vi "TLMB_Get_Single_Fault_Snapshot.vi"(0 "GEA2 Reference In":refnum<k24>, 5 "Standalone?":bool, 7 "Snapshot Selection":T2, 11 "Error In":errorcluster) -> (4 "GEA2 Reference Out":refnum<k24>, 6 "Fault Snapshots":T1, 15 "Error Out":errorcluster)   [LabVIEW 2021, in "TLMB.lvlib"]
uses:
  Projects/TLMB.lvlib
  subVIs/Snap_Selection.ctl
  D:/Common/LabVIEW GEA2 Toolkit/source/GEA3 DLL Source/GeaCommunication.dll
  Common/LabVIEW GEA2 Toolkit/source/GEA3 DLL Source/GeaCommunication.dll
  subVIs/Snap_Input.ctl
  Common/LabVIEW GEA2 Toolkit/GEA3/type defs/Source_Destination.ctl
  Common/LabVIEW GEA2 Toolkit/GEA3/type defs/ERD Read Data In.ctl
  Common/LabVIEW GEA2 Toolkit/GEA3/library/GEA2_Toolkit.lvlib
panel:
  out "ERD Number":string
  out "ERD Data":string
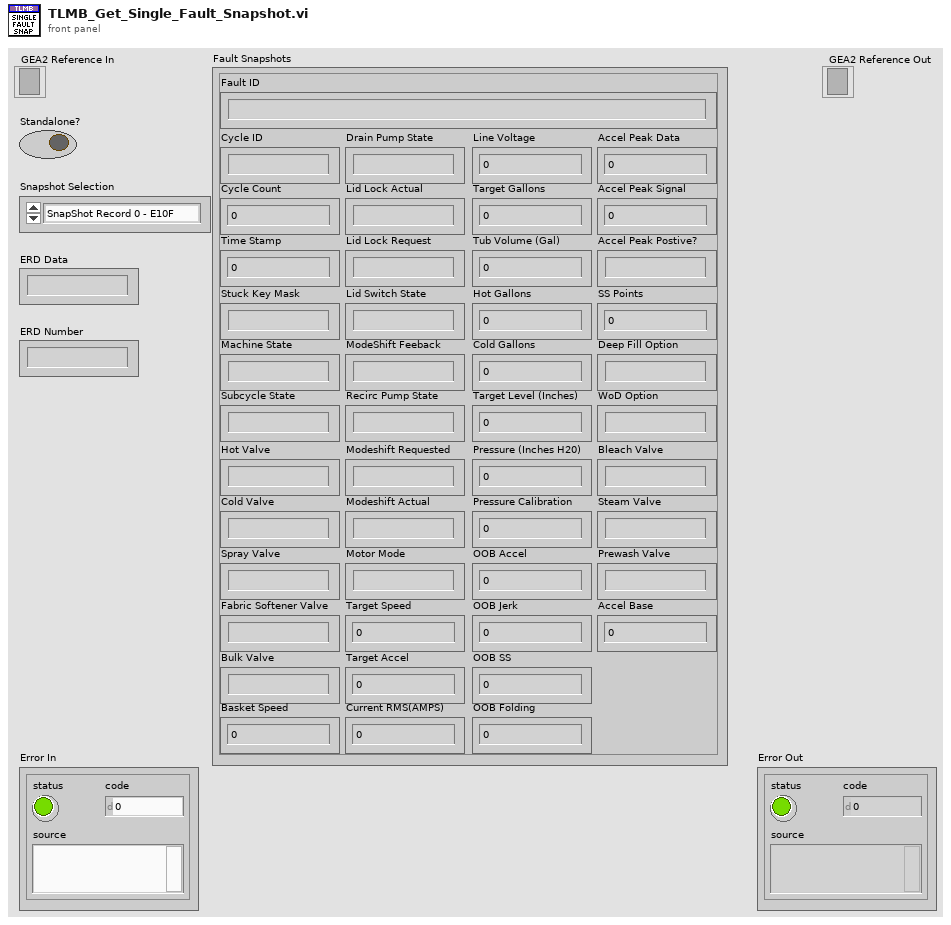
[diagram p1: front panel]
types:
  T1 = typedef "TLMB.lvlib/Snap_Input.ctl" = cluster{"Fault ID":string, "Cycle Count":u32, "Cycle ID":string, "Time Stamp":u32, "Stuck Key Mask":string, "Machine State":string, "Subcycle State":string, "Hot Valve":string, "Cold Valve":string, "Spray Valve":string, "Fabric Softener Valve":string, "Bulk Valve":string, "Drain Pump State":string, "Lid Lock Actual":string, "Lid Lock Request":string, "Lid Switch State":string, "ModeShift Feeback":string, "Recirc Pump State":string, "Modeshift Requested":string, "Modeshift Actual":string, "Motor Mode":string, "Target Speed":u16, "Target Accel":u16, "Current RMS(AMPS)":dbl, "Line Voltage":dbl, "Target Gallons":dbl, "Tub Volume (Gal)":dbl, "Hot Gallons":dbl, "Cold Gallons":dbl, "Target Level (Inches)":dbl, "Pressure (Inches H20) ":dbl, "Pressure Calibration":dbl, "OOB Accel":i32, "OOB Jerk":i32, "OOB SS":i32, "OOB Folding":i32, "Accel Peak Data":i16, "Accel Peak Signal":u8, "Accel Peak Postive?":string, "SS Points":u8, "Deep Fill Option":string, "WoD Option":string, "Basket Speed":u16, "Bleach Valve":string, "Steam Valve":string, "Prewash Valve":string, "Accel Base":i16}
  T2 = typedef "TLMB.lvlib/Snap_Selection.ctl" = enum16{"SnapShot Record 0 - E10F", "Snapshot Record 1 - E110", "Snapshot Record 2 - E111", "Snapshot Record 3 - E112", "Snapshot Record 4 - E113", "Snapshot Record 5 - E114", "Snapshot Record 6 - E115", "Snapshot Record 7 - E116", "Snapshot Record 8 - E117", "Snapshot Record 9 - E118"}
  T3 = typedef "Source_Destination.ctl" = cluster{"Source":u8, "Destination":u8}
  T4 = typedef "ERD Read Data In.ctl" = cluster{"ERD Number":u16, "Data Type":enum16{"string", "boolean", "uint8_t", "uint16_t", "uint32_t", "uint64_t", "int8_t", "int16_t", "int32_t", "int64_t"}}
  T5 = typedef "ERD Read Data Out.ctl" = cluster{"ERD Number":u16, "Data":string}
  T6 = cluster{"ERD Data Out[0]":T5, "ERD Data Out[1]":T5, "ERD Data Out[2]":T5, "ERD Data Out[3]":T5, "ERD Data Out[4]":T5, "ERD Data Out[5]":T5, "ERD Data Out[6]":T5, "ERD Data Out[7]":T5, "ERD Data Out[8]":T5}
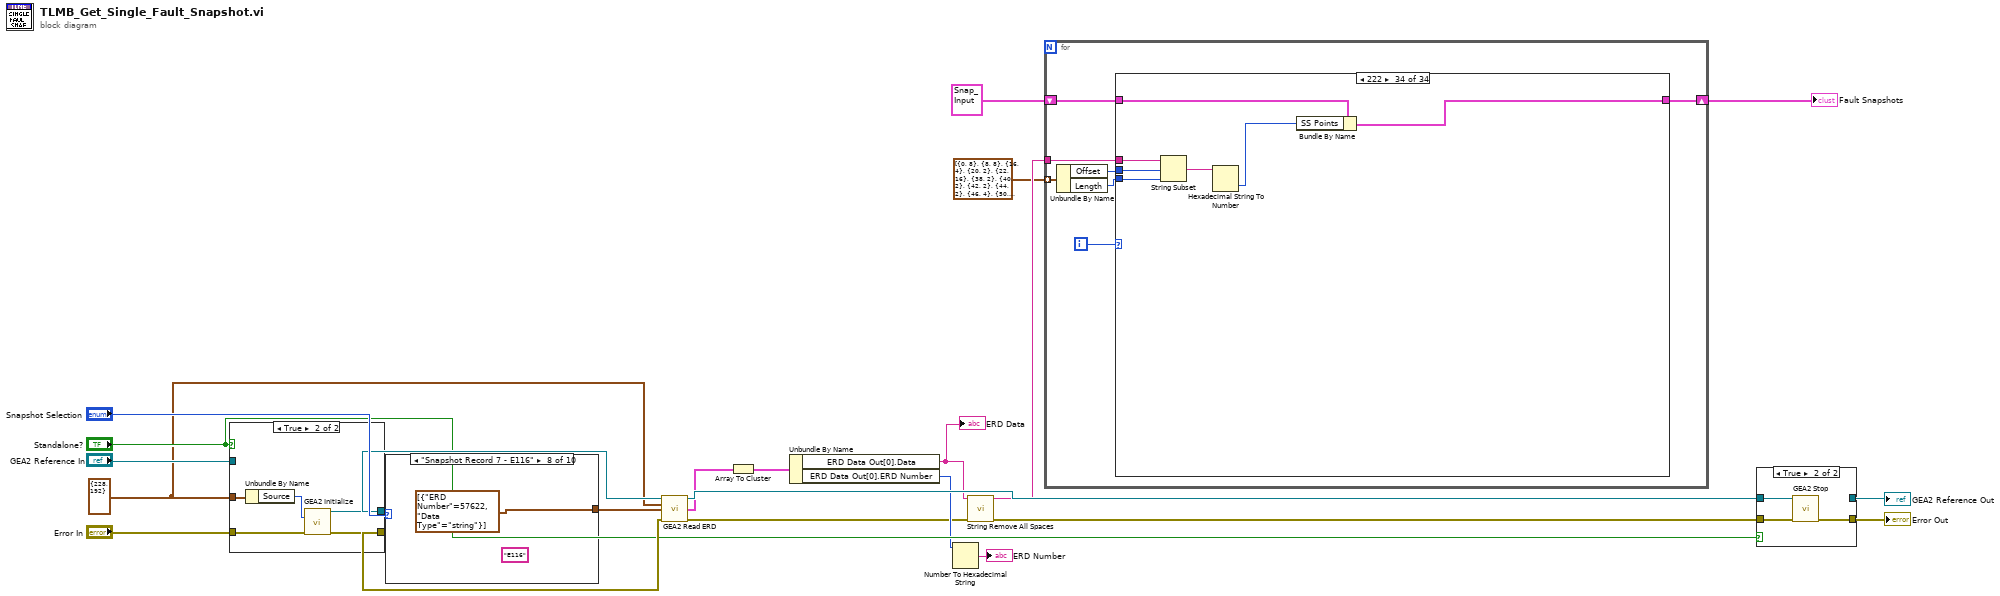
[diagram p0: block diagram]
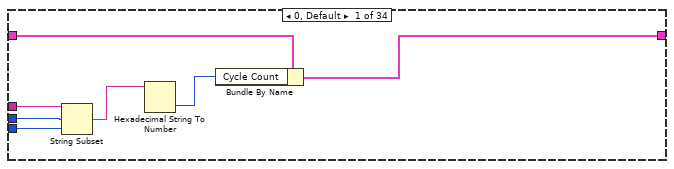
[diagram p2: hidden frame]
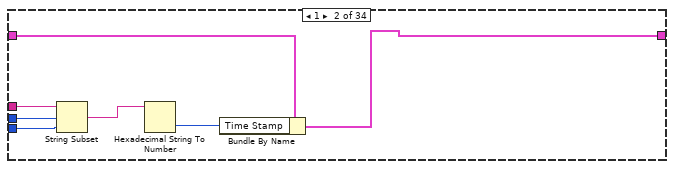
[diagram p3: hidden frame]
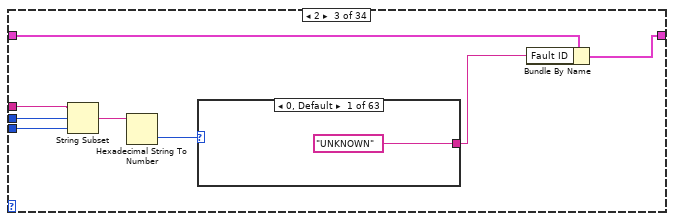
[diagram p4: hidden frame]
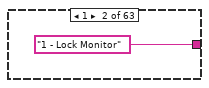
[diagram p5: hidden frame]
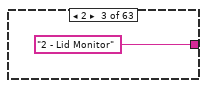
[diagram p6: hidden frame]
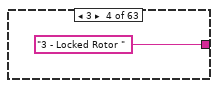
[diagram p7: hidden frame]
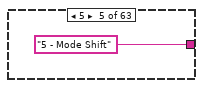
[diagram p8: hidden frame]
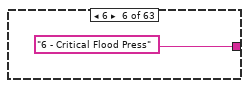
[diagram p9: hidden frame]
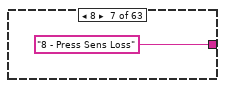
[diagram p10: hidden frame]
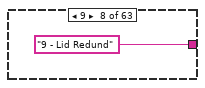
[diagram p11: hidden frame]
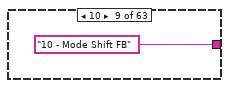
[diagram p12: hidden frame]
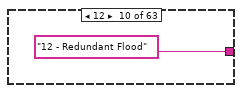
[diagram p13: hidden frame]
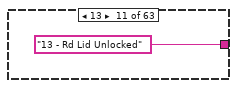
[diagram p14: hidden frame]
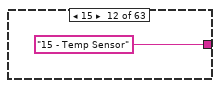
[diagram p15: hidden frame]
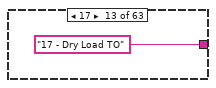
[diagram p16: hidden frame]
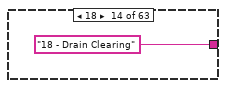
[diagram p17: hidden frame]
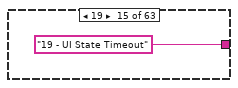
[diagram p18: hidden frame]
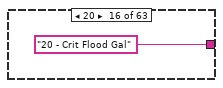
[diagram p19: hidden frame]
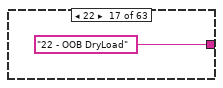
[diagram p20: hidden frame]
diagram:
  w13 = T3 {"Source"=228, "Destination"=192} ("GEA Inputs")
  n1 = case shown="True" "Standalone?" {
    tunnel: "Error In" -> [w23 w29]
    tunnel: [w23 w28] -> w17
    tunnel: "GEA2 Reference In" -> [w24 _]
    tunnel: [w24 w27] -> w18
    tunnel: w13 -> [_ w25]
    frame False {
    }
    frame True {
      n2 = Unbundle By Name(w25) -> ("Source"=w26:u8)
      n3 = call "GEA2 Initialize.vi"("Source Address"=w26, "error in"=w29) -> ("GEA2 Reference Out"=w27:refnum<k24>, "error out"=w28:errorcluster)  [unwired: 11 in, 1 out]
    }
  }
  n4 = case shown="\"Snapshot Record 7 - E116\"" "Snapshot Selection" {
    tunnel: [T4[] [{"ERD Number"=57615, "Data Type"=enum."string"}] ("Read ERD List") T4[] [{"ERD Number"=57616, "Data Type"=enum."string"}] ("Read ERD List") T4[] [{"ERD Number"=57617, "Data Type"=enum."string"}] ("Read ERD List") T4[] [{"ERD Number"=57618, "Data Type"=enum."string"}] ("Read ERD List") T4[] [{"ERD Number"=57619, "Data Type"=enum."string"}] ("Read ERD List") T4[] [{"ERD Number"=57620, "Data Type"=enum."string"}] ("Read ERD List") T4[] [{"ERD Number"=57621, "Data Type"=enum."string"}] ("Read ERD List") T4[] [{"ERD Number"=57622, "Data Type"=enum."string"}] ("Read ERD List") T4[] [{"ERD Number"=57623, "Data Type"=enum."string"}] ("Read ERD List") T4[] [{"ERD Number"=57624, "Data Type"=enum."string"}] ("Read ERD List")] -> w21
    frame "SnapShot Record 0 - E10F", Default {
      (unwired) "E10F"
    }
    frame "Snapshot Record 1 - E110" {
      (unwired) "E110"
    }
    frame "Snapshot Record 2 - E111" {
      (unwired) "E111"
    }
    frame "Snapshot Record 3 - E112" {
      (unwired) "E112"
    }
    frame "Snapshot Record 4 - E113" {
      (unwired) "E113"
    }
    frame "Snapshot Record 5 - E114" {
      (unwired) "E114"
    }
    frame "Snapshot Record 6 - E115" {
      (unwired) "E115"
    }
    frame "Snapshot Record 7 - E116" {
      (unwired) "E116"
    }
    frame "Snapshot Record 8 - E117" {
      (unwired) "E117"
    }
    frame "Snapshot Record 9 - E118" {
      (unwired) "E118"
    }
  }
  n5 = call "GEA2 Read ERD.vi"("GEA2 Reference In"=w18, "GEA Inputs"=w13, "Read ERD List"=w21, "Error In"=w17) -> ("GEA2 Reference Out"=w16:refnum<k24>, "ERD Data Out"=w12:T5[], "Error Out"=w7:errorcluster)  [unwired: 8 in, 1 out]
  n6 = Array To Cluster(array=w12) -> (cluster=w11:T6)
  n7 = Unbundle By Name(w11) -> ("ERD Data Out[0].Data"=w8:string, "ERD Data Out[0].ERD Number"=w10:u16)
  "ERD Data" <- w8
  n8 = Number To Hexadecimal String(2:w10) -> (0:→"ERD Number":string)  [unwired: 1 in]
  n9 = call "String Remove All Spaces.vi"("Input String"=w8, "error in (no error)"=w7) -> ("Spaces Removed"=w4:string, "error out"=w6:errorcluster)  [unwired: 12 in]
  n10 = for {
    tunnel: w4 -> [w46]
    shift-right: [w44] -> w1
    shift-left: T1 {"Fault ID"="", "Cycle Count"=0, "Cycle ID"="", "Time Stamp"=0, "Stuck Key Mask"="", "Machine State"="", "Subcycle State"="", "Hot Valve"="", "Cold Valve"="", "Spray Valve"="", "Fabric Softener Valve"="", "Bulk Valve"="", "Drain Pump State"="", "Lid Lock Actual"="", "Lid Lock Request"="", "Lid Switch State"="", "ModeShift Feeback"="", "Recirc Pump State"="", "Modeshift Requested"="", "Modeshift Actual"="", "Motor Mode"="", "Target Speed"=0, "Target Accel"=0, "Current RMS(AMPS)"=0.0, "Line Voltage"=0.0, "Target Gallons"=0.0, "Tub Volume (Gal)"=0.0, "Hot Gallons"=0.0, "Cold Gallons"=0.0, "Target Level (Inches)"=0.0, "Pressure (Inches H20) "=0.0, "Pressure Calibration"=0.0, "OOB Accel"=0, "OOB Jerk"=0, "OOB SS"=0, "OOB Folding"=0, "Accel Peak Data"=0, "Accel Peak Signal"=0, "Accel Peak Postive?"="", "SS Points"=0, "Deep Fill Option"="", "WoD Option"="", "Basket Speed"=0, "Bleach Valve"="", "Steam Valve"="", "Prewash Valve"="", "Accel Base"=0} ("input cluster") -> [w45]
    tunnel: cluster{"Offset":i32, "Length":i32}[] [{"Offset"=0, "Length"=8}, {"Offset"=8, "Length"=8}, {"Offset"=16, "Length"=4}, {"Offset"=20, "Length"=2}, {"Offset"=22, "Length"=16}, {"Offset"=38, "Length"=2}, {"Offset"=40, "Length"=2}, {"Offset"=42, "Length"=2}, {"Offset"=44, "Length"=2}, {"Offset"=46, "Length"=4}, {"Offset"=50, "Length"=4}, {"Offset"=54, "Length"=4}, {"Offset"=58, "Length"=4}, {"Offset"=62, "Length"=8}, {"Offset"=70, "Length"=8}, {"Offset"=78, "Length"=8}, {"Offset"=86, "Length"=8}, {"Offset"=94, "Length"=8}, {"Offset"=102, "Length"=8}, {"Offset"=110, "Length"=4}, {"Offset"=114, "Length"=2}, {"Offset"=116, "Length"=2}, {"Offset"=118, "Length"=4}, {"Offset"=104, "Length"=8}, {"Offset"=112, "Length"=8}, {"Offset"=120, "Length"=8}, {"Offset"=128, "Length"=8}, {"Offset"=136, "Length"=8}, {"Offset"=144, "Length"=4}, {"Offset"=148, "Length"=4}, {"Offset"=152, "Length"=2}, {"Offset"=154, "Length"=2}, {"Offset"=156, "Length"=2}, {"Offset"=158, "Length"=2}] -> [w41] mode=indexing
    i -> [w43]
    n11 = Unbundle By Name(w41) -> ("Offset"=w42:i32, "Length"=w40:i32)
    n12 = case shown="222" w43 {
      tunnel: w46 -> [w51 w60 w67 w139 w188 w211 w231 w264 w288 w301 w311 w321 w331 w341 w351 w358 w365 w372 w379 w386 w393 w401 w409 w420 w429 w448 w456 w464 w474 w484 w494 w520 w543 w557]
      tunnel: w42 -> [w50 w59 w66 w138 w187 w210 w230 w263 w287 w300 w310 w320 w330 w340 w350 w357 w364 w371 w378 w385 w392 w400 w408 w419 w428 w447 w455 w463 w473 w483 w493 w519 w542 w556]
      tunnel: w40 -> [w49 w58 w65 w137 w186 w209 w229 w262 w286 w299 w309 w319 w329 w339 w349 w356 w363 w370 w377 w384 w391 w399 w407 w418 w427 w446 w454 w462 w472 w482 w492 w518 w541 w555]
      tunnel: w45 -> [w53 w57 w68 w136 w190 w213 w228 w266 w290 w303 w313 w323 w333 w343 w353 w360 w367 w374 w381 w388 w395 w403 w412 w417 w431 w450 w458 w466 w476 w486 w496 w522 w545 w559]
      tunnel: [w52 w56 w64 w135 w189 w212 w227 w265 w289 w302 w312 w322 w332 w342 w352 w359 w366 w373 w380 w387 w394 w402 w411 w416 w430 w449 w457 w465 w475 w485 w495 w521 w544 w558] -> w44
      frame 0, Default {
        n13 = String Subset(string=w51, offset (0)=w50, length (rest)=w49) -> (substring=w48:string)
        n14 = Hexadecimal String To Number(string=w48) -> (number=w47:u32)  [unwired: 2 in, 1 out]
        n15 = Bundle By Name(cluster=w53, "Cycle Count"=w47) -> (w52:T1)
      }
      frame 1 {
        n16 = String Subset(string=w60, offset (0)=w59, length (rest)=w58) -> (substring=w55:string)
        n17 = Hexadecimal String To Number(string=w55) -> (number=w54:u32)  [unwired: 2 in, 1 out]
        n18 = Bundle By Name(cluster=w57, "Time Stamp"=w54) -> (w56:T1)
      }
      frame 2 {
        n19 = String Subset(string=w67, offset (0)=w66, length (rest)=w65) -> (substring=w63:string)
        n20 = Hexadecimal String To Number(string=w63) -> (number=w62:u32)  [unwired: 2 in, 1 out]
        n21 = case shown="0, Default" w62 {
          tunnel: ["UNKNOWN" "1 - Lock Monitor" "2 - Lid Monitor" "3 - Locked Rotor " "5 - Mode Shift" "6 - Critical Flood Press" "8 - Press Sens Loss" "9 - Lid Redund" "10 - Mode Shift FB" "12 - Redundant Flood" "13 - Rd Lid Unlocked" "15 - Temp Sensor" "17 - Dry Load TO" "18 - Drain Clearing" "19 - UI State Timeout" "20 - Crit Flood Gal" "22 - OOB DryLoad" "23 - Crit LidLock: Can't Lock" "24 - Lid Logic" "25 - Press Sens Dropout" "26 - OOB Redist" "27 - Water Access" "28 - ADC Knob" "29 - Suds Lock" "30 - Stuck Button" "31 - OOB Fallback" "32 - Crit LidLock: Can't Unlock" "33 - Crit Inv Reset in Run" "34 - Inv Boot Failure" "35 - Accel Chip Comm Failure" "41 - Inv LGBT Temp Sensor" "42 - Inv LGBT Temp Overheat" "43 - Inv Gate Driver" "44 - Inv Gate Crit Over Current" "45 - Inv DC Bus Voltage Crit" "46 - Inv MC API Ver" "47 - Inv MC Command Crit" "48 - Inv Heatsink Temp" "49 - Inv Motor Over Temp" "50 - Inv Crit Low Voltage" "51 - Inv Crit Locked Rotor" "52 - Inv Motor Over Temp" "100 - Accelrmtr Comm" "101 - Max Fill Pressure" "102 - Clock Mon" "103 - LidLock Failure" "104 - Adaptive Drain" "105 - Max Fill Volume" "106 - Target Spin Speed Timeout" "107 - Target Spin Speed Dropout" "108 - UI-MC Heatbeat Timeout" "109 - Event Seq Overflow" "111 - Inv Reset in Cycle Run" "114 - Utility Micro Comm" "115 - Accel Heartbeat" "119 - Inv LGBT Temp Overheat" "120 - Inv Gate Over Current" "121 - Inv DC Bus Voltage" "122 - Inv MC Command" "123 - Inv Heatsink Overheat" "124 - Inv Low Voltage" "125 - Inv Locked Rotor" "126 - Phase Fault"] -> w61
          frame 0, Default {
          }
          frame 1 {
          }
          frame 2 {
          }
          frame 3 {
          }
          frame 5 {
          }
          frame 6 {
          }
          frame 8 {
          }
          frame 9 {
          }
          frame 10 {
          }
          frame 12 {
          }
          frame 13 {
          }
          frame 15 {
          }
          frame 17 {
          }
          frame 18 {
          }
          frame 19 {
          }
          frame 20 {
          }
          frame 22 {
          }
          frame 23 {
          }
          frame 24 {
          }
          frame 25 {
          }
          frame 26 {
          }
          frame 27 {
          }
          frame 28 {
          }
          frame 29 {
          }
          frame 30 {
          }
          frame 31 {
          }
          frame 32 {
          }
          frame 33 {
          }
          frame 34 {
          }
          frame 35 {
          }
          frame 41 {
          }
          frame 42 {
          }
          frame 43 {
          }
          frame 44 {
          }
          frame 45 {
          }
          frame 46 {
          }
          frame 47 {
          }
          frame 48 {
          }
          frame 49 {
          }
          frame 50 {
          }
          frame 51 {
          }
          frame 52 {
          }
          frame 100 {
          }
          frame 101 {
          }
          frame 102 {
          }
          frame 103 {
          }
          frame 104 {
          }
          frame 105 {
          }
          frame 106 {
          }
          frame 107 {
          }
          frame 108 {
          }
          frame 109 {
          }
          frame 111 {
          }
          frame 114 {
          }
          frame 115 {
          }
          frame 119 {
          }
          frame 120 {
          }
          frame 121 {
          }
          frame 122 {
          }
          frame 123 {
          }
          frame 124 {
          }
          frame 125 {
          }
          frame 126 {
          }
        }
        n22 = Bundle By Name(cluster=w68, "Fault ID"=w61) -> (w64:T1)
      }
      frame 3 {
        n23 = String Subset(string=w139, offset (0)=w138, length (rest)=w137) -> (substring=w134:string)
        n24 = Hexadecimal String To Number(string=w134) -> (number=w133:u32)  [unwired: 2 in, 1 out]
        n25 = case shown="0, Default" w133 {
          tunnel: ["0 - NotDefined" "1 - BasketClean" "2 - DrainAndSpin" "3 - QuickRinse" "4 - BulkyItems" "5 - Sanitize" "6 - TowelsSheets" "8 - Normal_Mixedload" "9 - Whites" "10 - DarkColors" "11 - Jeans" "12 - HandWash" "13 - Delicates" "14 - SpeedWash" "15 - HeavyDuty" "16 - Allergen" "17 - PowerClean" "18 - RinseSpin" "19 - SingleItemWash" "20 - Colors" "21 - ColdWash" "22 - WaterOnDemand" "23 - TubClean" "24 - CasualsWithSteam" "25 - StainWashWithSteam" "26 - DeepClean" "27 - NotUsed_Start" "127 - NotUsed_End" "128 - Cottons" "129 - EasyCare" "130 - ActiveWear" "131 - TimedDry" "132 - DeWrinkle" "133 - QuickAirFluff" "134 - SteamRefresh" "135 - SteamDewrinkle" "136 - SpeedDry" "137 - Mixed" "138 - Quickdry" "139 - Casuals" "140 - Warmup" "141 - EnergySaver" "142 - Antibacterial"] -> w132
          frame 0, Default {
          }
          frame 1 {
          }
          frame 2 {
          }
          frame 3 {
          }
          frame 4 {
          }
          frame 5 {
          }
          frame 6 {
          }
          frame 8 {
          }
          frame 9 {
          }
          frame 10 {
          }
          frame 11 {
          }
          frame 12 {
          }
          frame 13 {
          }
          frame 14 {
          }
          frame 15 {
          }
          frame 16 {
          }
          frame 17 {
          }
          frame 18 {
          }
          frame 19 {
          }
          frame 20 {
          }
          frame 21 {
          }
          frame 22 {
          }
          frame 23 {
          }
          frame 24 {
          }
          frame 25 {
          }
          frame 26 {
          }
          frame 27 {
          }
          frame 127 {
          }
          frame 128 {
          }
          frame 129 {
          }
          frame 130 {
          }
          frame 131 {
          }
          frame 132 {
          }
          frame 133 {
          }
          frame 134 {
          }
          frame 135 {
          }
          frame 136 {
          }
          frame 137 {
          }
          frame 138 {
          }
          frame 139 {
          }
          frame 140 {
          }
          frame 141 {
          }
          frame 142 {
          }
        }
        n26 = Bundle By Name(cluster=w136, "Cycle ID"=w132) -> (w135:T1)
      }
      frame 4 {
        (unwired) ""
        n27 = String Subset(string=w188, offset (0)=w187, length (rest)=w186) -> (substring=w185:string)
        n28 = Hexadecimal String To Number(string=w185) -> (number=w184:u32)  [unwired: 2 in, 1 out]
        n29 = case shown="0, Default" w184 {
          tunnel: ["No Stuck Key" "Smart Dispense" "Delay Wash" "Extra Rinse" "Mycycle" "Spin Button" "Deep Rinse" "Soil Button" "Auto Soak" "Temp Button" "Warm Rinse" "Deep Fill" "Water on Demand" "Power Button" "Start Button"] -> w183
          frame 0, Default {
          }
          frame 1 {
          }
          frame 2 {
          }
          frame 4 {
          }
          frame 8 {
          }
          frame 16 {
          }
          frame 32 {
          }
          frame 64 {
          }
          frame 128 {
          }
          frame 256 {
          }
          frame 512 {
          }
          frame 1024 {
          }
          frame 2048 {
          }
          frame 4096 {
          }
          frame 8192 {
          }
        }
        n30 = Bundle By Name(cluster=w190, "Stuck Key Mask"=w183) -> (w189:T1)
      }
      frame 5 {
        n31 = String Subset(string=w211, offset (0)=w210, length (rest)=w209) -> (substring=w208:string)
        n32 = Hexadecimal String To Number(string=w208) -> (number=w207:u32)  [unwired: 2 in, 1 out]
        n33 = case shown="0, Default" w207 {
          tunnel: ["IDLE" "STANDBY" "RUN" "PAUSE" "EOC" "DSM DELAY RUN" "DELAY RUN" "DELAY PAUSE" "DRAIN TIMEOUT" "CLEAN SPEAK"] -> w206
          frame 0, Default {
          }
          frame 1 {
          }
          frame 2 {
          }
          frame 3 {
          }
          frame 4 {
          }
          frame 5 {
          }
          frame 6 {
          }
          frame 7 {
          }
          frame 8 {
          }
          frame 128 {
          }
        }
        n34 = Bundle By Name(cluster=w213, "Machine State"=w206) -> (w212:T1)
      }
      frame 6 {
        n35 = String Subset(string=w231, offset (0)=w230, length (rest)=w229) -> (substring=w226:string)
        n36 = Hexadecimal String To Number(string=w226) -> (number=w225:u32)  [unwired: 2 in, 1 out]
        n37 = case shown="0, Default" w225 {
          tunnel: ["NONE" "FILL" "SOAK" "WASH" "RINSE" "SPIN" "DRAIN" "EXTRA SPIN" "EXTRA RINSE" "TUMBLE" "LOAD SIZE"] -> w224
          frame 0, Default {
          }
          frame 1 {
          }
          frame 2 {
          }
          frame 3 {
          }
          frame 4 {
          }
          frame 5 {
          }
          frame 6 {
          }
          frame 7 {
          }
          frame 8 {
          }
          frame 9 {
          }
          frame 10 {
          }
        }
        n38 = Bundle By Name(cluster=w228, "Subcycle State"=w224) -> (w227:T1)
      }
      frame 7 {
        n39 = String Subset(string=w264, offset (0)=w263, length (rest)=w262) -> (substring=w260:string)
        n40 = Hexadecimal String To Number(string=w260) -> (number=w261:u32)  [unwired: 2 in, 1 out]
        n41 = Number To Boolean Array(number=w261) -> (Boolean array=w259:bool[])
        n42 = Index Array(array=w259) -> (element #1=w258:bool, element #2=w256:bool, element #3=w255:bool, element #4=w254:bool, element #5=w253:bool, element #6=w245:bool, element #7=w244:bool, element #8=w243:bool)  [unwired: 8 in]
        n43 = case shown="False" w258 {
          tunnel: ["OFF" "ON"] -> w257
          frame False {
          }
          frame True {
          }
        }
        n44 = case shown="False" w256 {
          tunnel: ["OFF" "ON"] -> w252
          frame False {
          }
          frame True {
          }
        }
        n45 = case shown="False" w255 {
          tunnel: ["OFF" "ON"] -> w251
          frame False {
          }
          frame True {
          }
        }
        n46 = case shown="False" w254 {
          tunnel: ["OFF" "ON"] -> w250
          frame False {
          }
          frame True {
          }
        }
        n47 = case shown="False" w253 {
          tunnel: ["OFF" "ON"] -> w249
          frame False {
          }
          frame True {
          }
        }
        n48 = case shown="False" w245 {
          tunnel: ["OFF" "ON"] -> w248
          frame False {
          }
          frame True {
          }
        }
        n49 = case shown="False" w244 {
          tunnel: ["OFF" "ON"] -> w247
          frame False {
          }
          frame True {
          }
        }
        n50 = case shown="False" w243 {
          tunnel: ["OFF" "ON"] -> w246
          frame False {
          }
          frame True {
          }
        }
        n51 = Bundle By Name(cluster=w266, "Hot Valve"=w257, "Cold Valve"=w252, "Spray Valve"=w251, "Fabric Softener Valve"=w250, "Bulk Valve"=w249, "Bleach Valve"=w248, "Steam Valve"=w247, "Prewash Valve"=w246) -> (w265:T1)
      }
      frame 8 {
        n52 = String Subset(string=w288, offset (0)=w287, length (rest)=w286) -> (substring=w285:string)
        n53 = Hexadecimal String To Number(string=w285) -> (number=w284:u32)  [unwired: 2 in, 1 out]
        n54 = case shown="4" w284 {
          tunnel: ["UNKNOWN" "AGITATE" "SPIN" "TRANS TO SPIN" "TRANS TO AGITATE"] -> w283
          frame 0, Default {
          }
          frame 1 {
          }
          frame 2 {
          }
          frame 3 {
          }
          frame 4 {
          }
        }
        n55 = Bundle By Name(cluster=w290, "Modeshift Actual"=w283) -> (w289:T1)
      }
      frame 9 {
        n56 = String Subset(string=w301, offset (0)=w300, length (rest)=w299) -> (substring=w298:string)
        n57 = Hexadecimal String To Number(string=w298) -> (number=w297:u32)  [unwired: 2 in, 1 out]
        n58 = To Unsigned Word Integer(number=w297) -> (unsigned 16bit integer=w296:u16)
        n59 = Bundle By Name(cluster=w303, "Basket Speed"=w296) -> (w302:T1)
      }
      frame 10 {
        n60 = String Subset(string=w311, offset (0)=w310, length (rest)=w309) -> (substring=w308:string)
        n61 = Hexadecimal String To Number(string=w308) -> (number=w305:u32)  [unwired: 2 in, 1 out]
        n62 = To Double Precision Float(number=w305) -> (double precision float=w307:dbl)
        n63 = Divide(x=w307, y=100.0) -> (x/y=w304:dbl)
        n64 = Bundle By Name(cluster=w313, "Tub Volume (Gal)"=w304) -> (w312:T1)
      }
      frame 11 {
        n65 = String Subset(string=w321, offset (0)=w320, length (rest)=w319) -> (substring=w318:string)
        n66 = Hexadecimal String To Number(string=w318) -> (number=w315:u32)  [unwired: 2 in, 1 out]
        n67 = To Double Precision Float(number=w315) -> (double precision float=w317:dbl)
        n68 = Divide(x=w317, y=100.0) -> (x/y=w314:dbl)
        n69 = Bundle By Name(cluster=w323, "Hot Gallons"=w314) -> (w322:T1)
      }
      frame 12 {
        n70 = String Subset(string=w331, offset (0)=w330, length (rest)=w329) -> (substring=w328:string)
        n71 = Hexadecimal String To Number(string=w328) -> (number=w325:u32)  [unwired: 2 in, 1 out]
        n72 = To Double Precision Float(number=w325) -> (double precision float=w327:dbl)
        n73 = Divide(x=w327, y=100.0) -> (x/y=w324:dbl)
        n74 = Bundle By Name(cluster=w333, "Cold Gallons"=w324) -> (w332:T1)
      }
      frame 13 {
        n75 = String Subset(string=w341, offset (0)=w340, length (rest)=w339) -> (substring=w338:string)
        n76 = Hexadecimal String To Number(string=w338) -> (number=w335:u32)  [unwired: 2 in, 1 out]
        n77 = To Double Precision Float(number=w335) -> (double precision float=w337:dbl)
        n78 = Divide(x=w337, y=1000.0) -> (x/y=w334:dbl)
        n79 = Bundle By Name(cluster=w343, "Pressure (Inches H20)"=w334) -> (w342:T1)
      }
      frame 14 {
        n80 = String Subset(string=w351, offset (0)=w350, length (rest)=w349) -> (substring=w348:string)
        n81 = Hexadecimal String To Number(string=w348) -> (number=w345:u32)  [unwired: 2 in, 1 out]
        n82 = To Double Precision Float(number=w345) -> (double precision float=w347:dbl)
        n83 = Divide(x=w347, y=1000.0) -> (x/y=w344:dbl)
        n84 = Bundle By Name(cluster=w353, "Pressure Calibration"=w344) -> (w352:T1)
      }
      frame 15 {
        n85 = String Subset(string=w358, offset (0)=w357, length (rest)=w356) -> (substring=w355:string)
        n86 = Hexadecimal String To Number(string=w355) -> (number=w354:u32)  [unwired: 2 in, 1 out]
        n87 = Bundle By Name(cluster=w360, "OOB Accel"=w354) -> (w359:T1)
      }
      frame 16 {
        n88 = String Subset(string=w365, offset (0)=w364, length (rest)=w363) -> (substring=w362:string)
        n89 = Hexadecimal String To Number(string=w362) -> (number=w361:u32)  [unwired: 2 in, 1 out]
        n90 = Bundle By Name(cluster=w367, "OOB Jerk"=w361) -> (w366:T1)
      }
      frame 17 {
        n91 = String Subset(string=w372, offset (0)=w371, length (rest)=w370) -> (substring=w369:string)
        n92 = Hexadecimal String To Number(string=w369) -> (number=w368:u32)  [unwired: 2 in, 1 out]
        n93 = Bundle By Name(cluster=w374, "OOB SS"=w368) -> (w373:T1)
      }
      frame 18 {
        n94 = String Subset(string=w379, offset (0)=w378, length (rest)=w377) -> (substring=w376:string)
        n95 = Hexadecimal String To Number(string=w376) -> (number=w375:u32)  [unwired: 2 in, 1 out]
        n96 = Bundle By Name(cluster=w381, "OOB Folding"=w375) -> (w380:T1)
      }
      frame 19 {
        n97 = String Subset(string=w386, offset (0)=w385, length (rest)=w384) -> (substring=w383:string)
        n98 = Hexadecimal String To Number(string=w383) -> (number=w382:u32)  [unwired: 2 in, 1 out]
        n99 = Bundle By Name(cluster=w388, "Accel Peak Data"=w382) -> (w387:T1)
      }
      frame 20 {
        n100 = String Subset(string=w393, offset (0)=w392, length (rest)=w391) -> (substring=w390:string)
        n101 = Hexadecimal String To Number(string=w390) -> (number=w389:u32)  [unwired: 2 in, 1 out]
        n102 = Bundle By Name(cluster=w395, "Accel Peak Signal"=w389) -> (w394:T1)
      }
      frame 21 {
        n103 = String Subset(string=w401, offset (0)=w400, length (rest)=w399) -> (substring=w398:string)
        n104 = Hexadecimal String To Number(string=w398) -> (number=w397:u32)  [unwired: 2 in, 1 out]
        n105 = case shown="1" w397 {
          tunnel: ["FALSE" "TRUE"] -> w396
          frame 0, Default {
          }
          frame 1 {
          }
        }
        n106 = Bundle By Name(cluster=w403, "Accel Peak Postive?"=w396) -> (w402:T1)
      }
      frame 22 {
        n107 = String Subset(string=w409, offset (0)=w408, length (rest)=w407) -> (substring=w410:string)
        n108 = Hexadecimal String To Number(string=w410) -> (number=w406:u32)  [unwired: 2 in, 1 out]
        n109 = Bundle By Name(cluster=w412, "Accel Base"=w406) -> (w411:T1)
      }
      frame 23 {
        n110 = String Subset(string=w420, offset (0)=w419, length (rest)=w418) -> (substring=w415:string)
        n111 = Hexadecimal String To Number(string=w415) -> (number=w414:u32)  [unwired: 2 in, 1 out]
        n112 = case shown="0, Default" w414 {
          tunnel: ["0 - Deep Fill Off" "1 - Deep Fill On" "2 - Deep Fill Max"] -> w413
          frame 0, Default {
          }
          frame 1 {
          }
          frame 2 {
          }
        }
        n113 = Bundle By Name(cluster=w417, "Deep Fill Option"=w413) -> (w416:T1)
      }
      frame 24 {
        n114 = String Subset(string=w429, offset (0)=w428, length (rest)=w427) -> (substring=w426:string)
        n115 = Hexadecimal String To Number(string=w426) -> (number=w425:u32)  [unwired: 2 in, 1 out]
        n116 = case shown="0, Default" w425 {
          tunnel: ["IDLE" "FILL ACTIVE" "FILL PENDING" "FILL PAUSED" "FILL SOAK" "FULL" "DISARM SELECT" "DISARM DESELECT" "DRAINING"] -> w424
          frame 0, Default {
          }
          frame 1 {
          }
          frame 2 {
          }
          frame 3 {
          }
          frame 4 {
          }
          frame 5 {
          }
          frame 6 {
          }
          frame 7 {
          }
          frame 8 {
          }
        }
        n117 = Bundle By Name(cluster=w431, "WoD Option"=w424) -> (w430:T1)
      }
      frame 25 {
        n118 = String Subset(string=w448, offset (0)=w447, length (rest)=w446) -> (substring=w445:string)
        n119 = Hexadecimal String To Number(string=w445) -> (number=w442:u32)  [unwired: 2 in, 1 out]
        n120 = To Double Precision Float(number=w442) -> (double precision float=w444:dbl)
        n121 = Divide(x=w444, y=1000.0) -> (x/y=w441:dbl)
        n122 = Bundle By Name(cluster=w450, "Target Level (Inches)"=w441) -> (w449:T1)
      }
      frame 26 {
        n123 = String Subset(string=w456, offset (0)=w455, length (rest)=w454) -> (substring=w453:string)
        n124 = Hexadecimal String To Number(string=w453) -> (number=w452:u32)  [unwired: 2 in, 1 out]
        n125 = To Unsigned Word Integer(number=w452) -> (unsigned 16bit integer=w451:u16)
        n126 = Bundle By Name(cluster=w458, "Target Speed"=w451) -> (w457:T1)
      }
      frame 27 {
        n127 = String Subset(string=w464, offset (0)=w463, length (rest)=w462) -> (substring=w461:string)
        n128 = Hexadecimal String To Number(string=w461) -> (number=w460:u32)  [unwired: 2 in, 1 out]
        n129 = To Unsigned Word Integer(number=w460) -> (unsigned 16bit integer=w459:u16)
        n130 = Bundle By Name(cluster=w466, "Target Accel"=w459) -> (w465:T1)
      }
      frame 28 {
        n131 = String Subset(string=w474, offset (0)=w473, length (rest)=w472) -> (substring=w471:string)
        n132 = Hexadecimal String To Number(string=w471) -> (number=w470:u32)  [unwired: 2 in, 1 out]
        n133 = To Double Precision Float(number=w470) -> (double precision float=w469:dbl)
        n134 = Divide(x=w469, y=1024.0) -> (x/y=w467:dbl)
        n135 = Bundle By Name(cluster=w476, "Current RMS(AMPS)"=w467) -> (w475:T1)
      }
      frame 29 {
        n136 = String Subset(string=w484, offset (0)=w483, length (rest)=w482) -> (substring=w481:string)
        n137 = Hexadecimal String To Number(string=w481) -> (number=w480:u32)  [unwired: 2 in, 1 out]
        n138 = To Double Precision Float(number=w480) -> (double precision float=w479:dbl)
        n139 = Divide(x=w479, y=32.0) -> (x/y=w477:dbl)
        n140 = Bundle By Name(cluster=w486, "Line Voltage"=w477) -> (w485:T1)
      }
      frame 30 {
        n141 = String Subset(string=w494, offset (0)=w493, length (rest)=w492) -> (substring=w491:string)
        n142 = Hexadecimal String To Number(string=w491) -> (number=w488:u32)  [unwired: 2 in, 1 out]
        n143 = To Double Precision Float(number=w488) -> (double precision float=w490:dbl)
        n144 = Divide(x=w490, y=100.0) -> (x/y=w487:dbl)
        n145 = Bundle By Name(cluster=w496, "Target Gallons"=w487) -> (w495:T1)
      }
      frame 999 {
        n146 = String Subset(string=w520, offset (0)=w519, length (rest)=w518) -> (substring=w517:string)
        n147 = Hexadecimal String To Number(string=w517) -> (number=w516:u32)  [unwired: 2 in, 1 out]
        n148 = Number To Boolean Array(number=w516) -> (Boolean array=w515:bool[])
        n149 = Index Array(array=w515) -> (element #1=w513:bool, element #2=w512:bool, element #3=w509:bool, element #4=w508:bool, element #5=w505:bool, element #6=w504:bool, element #7=w502:bool, element #8=w501:bool)  [unwired: 8 in]
        n150 = Boolean To (0,1)(Boolean=w502) -> (0, 1=w499:i16)
        n151 = Boolean To (0,1)(Boolean=w501) -> (0, 1=w500:i16)
        n152 = Add(x=w499, y=w500) -> (x+y=w498:i16)
        n153 = case shown="True" w505 {
          tunnel: ["AGITATE" "SPIN"] -> w506
          frame False {
          }
          frame True {
          }
        }
        n154 = case shown="True" w504 {
          tunnel: ["OFF" "ON"] -> w503
          frame False {
          }
          frame True {
          }
        }
        n155 = case shown="True" w513 {
          tunnel: ["OFF" "ON"] -> w514
          frame False {
          }
          frame True {
          }
        }
        n156 = case shown="True" w512 {
          tunnel: ["UNLOCKED" "LOCKED"] -> w511
          frame False {
          }
          frame True {
          }
        }
        n157 = case shown="True" w509 {
          tunnel: ["UNLOCKED" "LOCKED"] -> w510
          frame False {
          }
          frame True {
          }
        }
        n158 = case shown="True" w508 {
          tunnel: ["OPEN" "CLOSED"] -> w507
          frame False {
          }
          frame True {
          }
        }
        n159 = case shown="2" w498 {
          tunnel: ["UNKNOWN" "AGITATE" "SPIN"] -> w497
          frame 0, Default {
          }
          frame 1 {
          }
          frame 2 {
          }
        }
        n160 = Bundle By Name(cluster=w522, "Drain Pump State"=w514, "Lid Lock Actual"=w511, "Lid Lock Request"=w510, "Lid Switch State"=w507, "ModeShift Feeback"=w506, "Recirc Pump State"=w503, "Modeshift Requested"=w497) -> (w521:T1)
      }
      frame 1111 {
        n161 = String Subset(string=w543, offset (0)=w542, length (rest)=w541) -> (substring=w540:string)
        n162 = Hexadecimal String To Number(string=w540) -> (number=w539:u32)  [unwired: 2 in, 1 out]
        n163 = case shown="0, Default" w539 {
          tunnel: ["CLOSED LOOP" "CLOSED LOOP ANGLE" "OPEN LOOP" "OPEN LOOP ANGLE" "COASTING" "BRAKING" "IDLE"] -> w538
          frame 0, Default {
          }
          frame 1 {
          }
          frame 2 {
          }
          frame 3 {
          }
          frame 4 {
          }
          frame 5 {
          }
          frame 6 {
          }
        }
        n164 = Bundle By Name(cluster=w545, "Motor Mode"=w538) -> (w544:T1)
      }
      frame 222 {
        n165 = String Subset(string=w557, offset (0)=w556, length (rest)=w555) -> (substring=w554:string)
        n166 = Hexadecimal String To Number(string=w554) -> (number=w553:u32)  [unwired: 2 in, 1 out]
        n167 = Bundle By Name(cluster=w559, "SS Points"=w553) -> (w558:T1)
      }
    }
  }
  "Fault Snapshots" <- w1
  n168 = case shown="True" "Standalone?" {
    tunnel: [w560 w564] -> w5
    tunnel: w16 -> [w561 w563]
    tunnel: [w561 _] -> w15
    tunnel: w6 -> [w560 w562]
    frame False {
    }
    frame True {
      n169 = call "GEA2 Stop.vi"("GEA2 Reference In"=w563, "Error In"=w562) -> ("Error Out"=w564:errorcluster)  [unwired: 13 in]
    }
  }
  "GEA2 Reference Out" <- w15
  "Error Out" <- w5
